vi "Trigger_CereStim_During_ PAL_Task.vi"() -> ()   [LabVIEW 2024]
uses:
  <vilib>/DAQmx/write.llb/DAQmx Write (Analog DBL 1Chan 1Samp).vi
  <vilib>/DAQmx/read.llb/DAQmx Read (Analog 1D Wfm NChan 1Samp).vi
  <vilib>/DAQmx/create/channels.llb/DAQmx Create Channel (AI-Voltage-Basic).vi
  <vilib>/DAQmx/create/channels.llb/DAQmx Create Channel (AO-Voltage-Basic).vi
  <vilib>/DAQmx/miscellaneous.llb/DAQmx Fill In Error Info.vi
  <vilib>/measure/mamon.llb/Trigger Detection for 1 Channel.vi
  <vilib>/measure/NI_MAPro.lvlib
panel:
  in  "Stimulation Offset\n(only for cond 10)":dbl=1.0
  out "Last STIMULATION ON Time":timestamp format="%<%.6X\n%x>T"
  in  "Acquisition Fs":i32=200
  in  "STIM 1 On 1 OFF":bool=TRUE
  out "Stimulation Pulse Counter":u64
  in  "Stimulation TTL Freq":dbl=50.0
  out "Reinforcement Threshold For Correct Incorrect":dbl
  in  "Reinforcement Signal Duration\nFor Incorrect":dbl=0.1
  in  "Reinforcement Signal Duration\nFor correct":dbl=0.07
  in  "Hysthersis":dbl=0.1
  in  "Event Detection Threshold (V)":dbl=3.0
  out "% NoSTIM Success":dbl format="%2_2g"
  out "#Success: NoSTIM":u32
  out "# Trials: NoSTIM":u32
  out "% STIM Success":dbl format="%2_2g"
  out "# Success: STIM":u32
  out "# Trials: STIM":u32
  out "% Success":dbl format="%2_2g"
  out "# Success":u32
  in  "Set StimulationManually, ALWAYS:":bool=TRUE
  in  "Manually Control Stimulation":bool=TRUE
  out "Trial Structure":string[](array[string])
  in  "Stimulation Probability":dbl=0.5 min=0.05 max=0.95 step=0.1
  out "Stimulation ON?":bool
  out "Time Elapsed since last event Offset":dbl
  out "Time Elapsed Since last trial":dbl
  out "Last STIMULUSINFO OFF":timestamp format="%<%.6X\n%x>T"
  out "Time Last Reinforcement":timestamp format="%<%.6X\n%x>T"
  out "Last Trial End":timestamp format="%<%.6X\n%x>T"
  out "Stimulation Trial":bool
  in  "Stimulation Onset time (Before each event )":dbl=2.0
  out "# Trials":u32
  out "Previous Trial: Correct/Incorrect":bool
  in  "STIMULATION CONDITION":u16(ring)=4 items=["--NONE SELECTED--", "1 Pre Sample Onset (STOPS AT STIMULUSINFO OFF)", "2 Pre Choice Onset (STOPS AT STIMULUSINFO OFF)", "3 Pre Sample And Choice Onset (STOPS AT STIMULUSINFO OFF)", "4 Pre 1st Sample till SamplePhase Offset ", "5 Pre 1st Choice till ChoicePhase Offset ", "6 During MemoryDelay  (NO STIMULATION ONSET TIME)", "7 During ITI (NO STIMULATION ONSET TIME)", "8 Entire Trial (Starts Pre 1st Sample ends at trial end)", "*9 Pre Sample Onset (STOPS AT STIMULUSINFO ON)", "10 PreStim(n-m seconds)"]
  out "ReinfoDur":dbl format="%_4g"
  out "TIME Reinforcement OFF":timestamp format="%<%.6X\n%x>T"
  out "TIME Reinforcement ON":timestamp format="%<%.6X\n%x>T"
  out "REINFORCEMENTINFO \nOFF Count":u32
  out "REINFORCEMENTINFO \nON Count":u32
  out "STIMULUSINFO \nOFF Count":u32
  out "STIMULUSINFO \nON Count":u32
  in  "stop":bool
  in  "Punishment Dur":dbl=7.0
  in  "Pump Dur":dbl=2.0
  in  "Memory Delay":dbl=7.0
  in  "Stimulation Fs":i32=1000
  in  "ITI":dbl=5.0
  in  "PAL TASK":u16=4
  in  "ICI":dbl=4.0
  in  "ISI":dbl=3.0
  # "PAL TASK"
  # "Tracking timings and events"
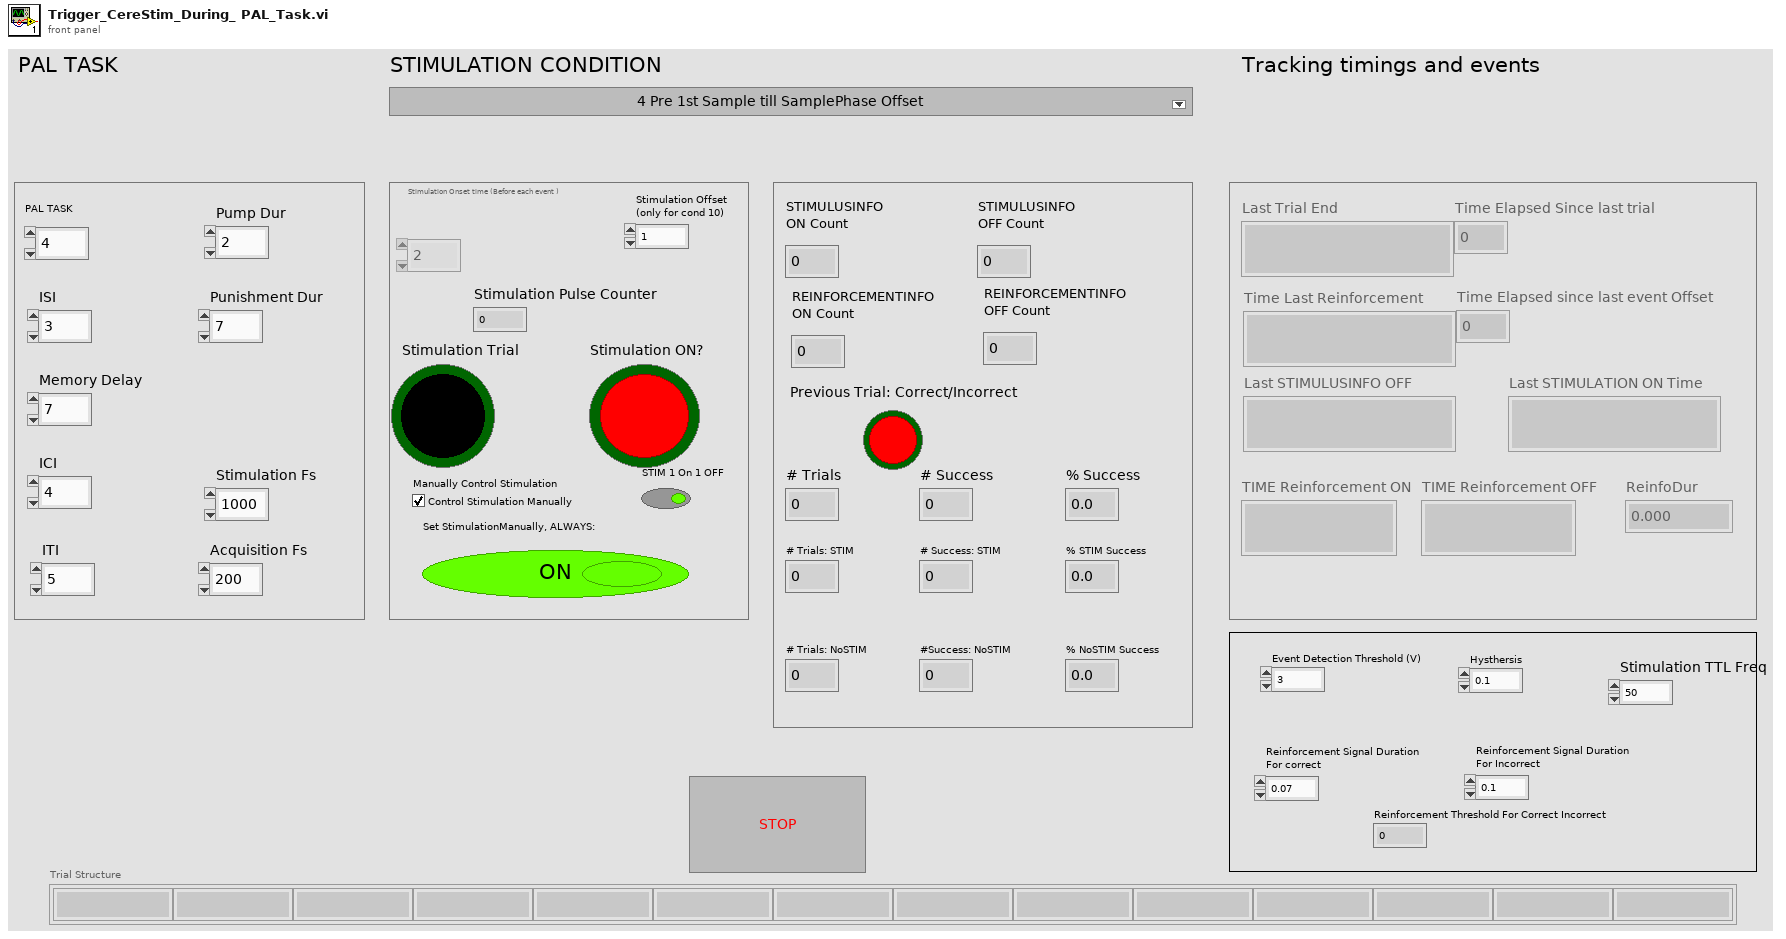
[diagram p1: front panel]
types:
  T1 = enum8{"Enabled", "Disabled", "Disabled and Grayed Out"}
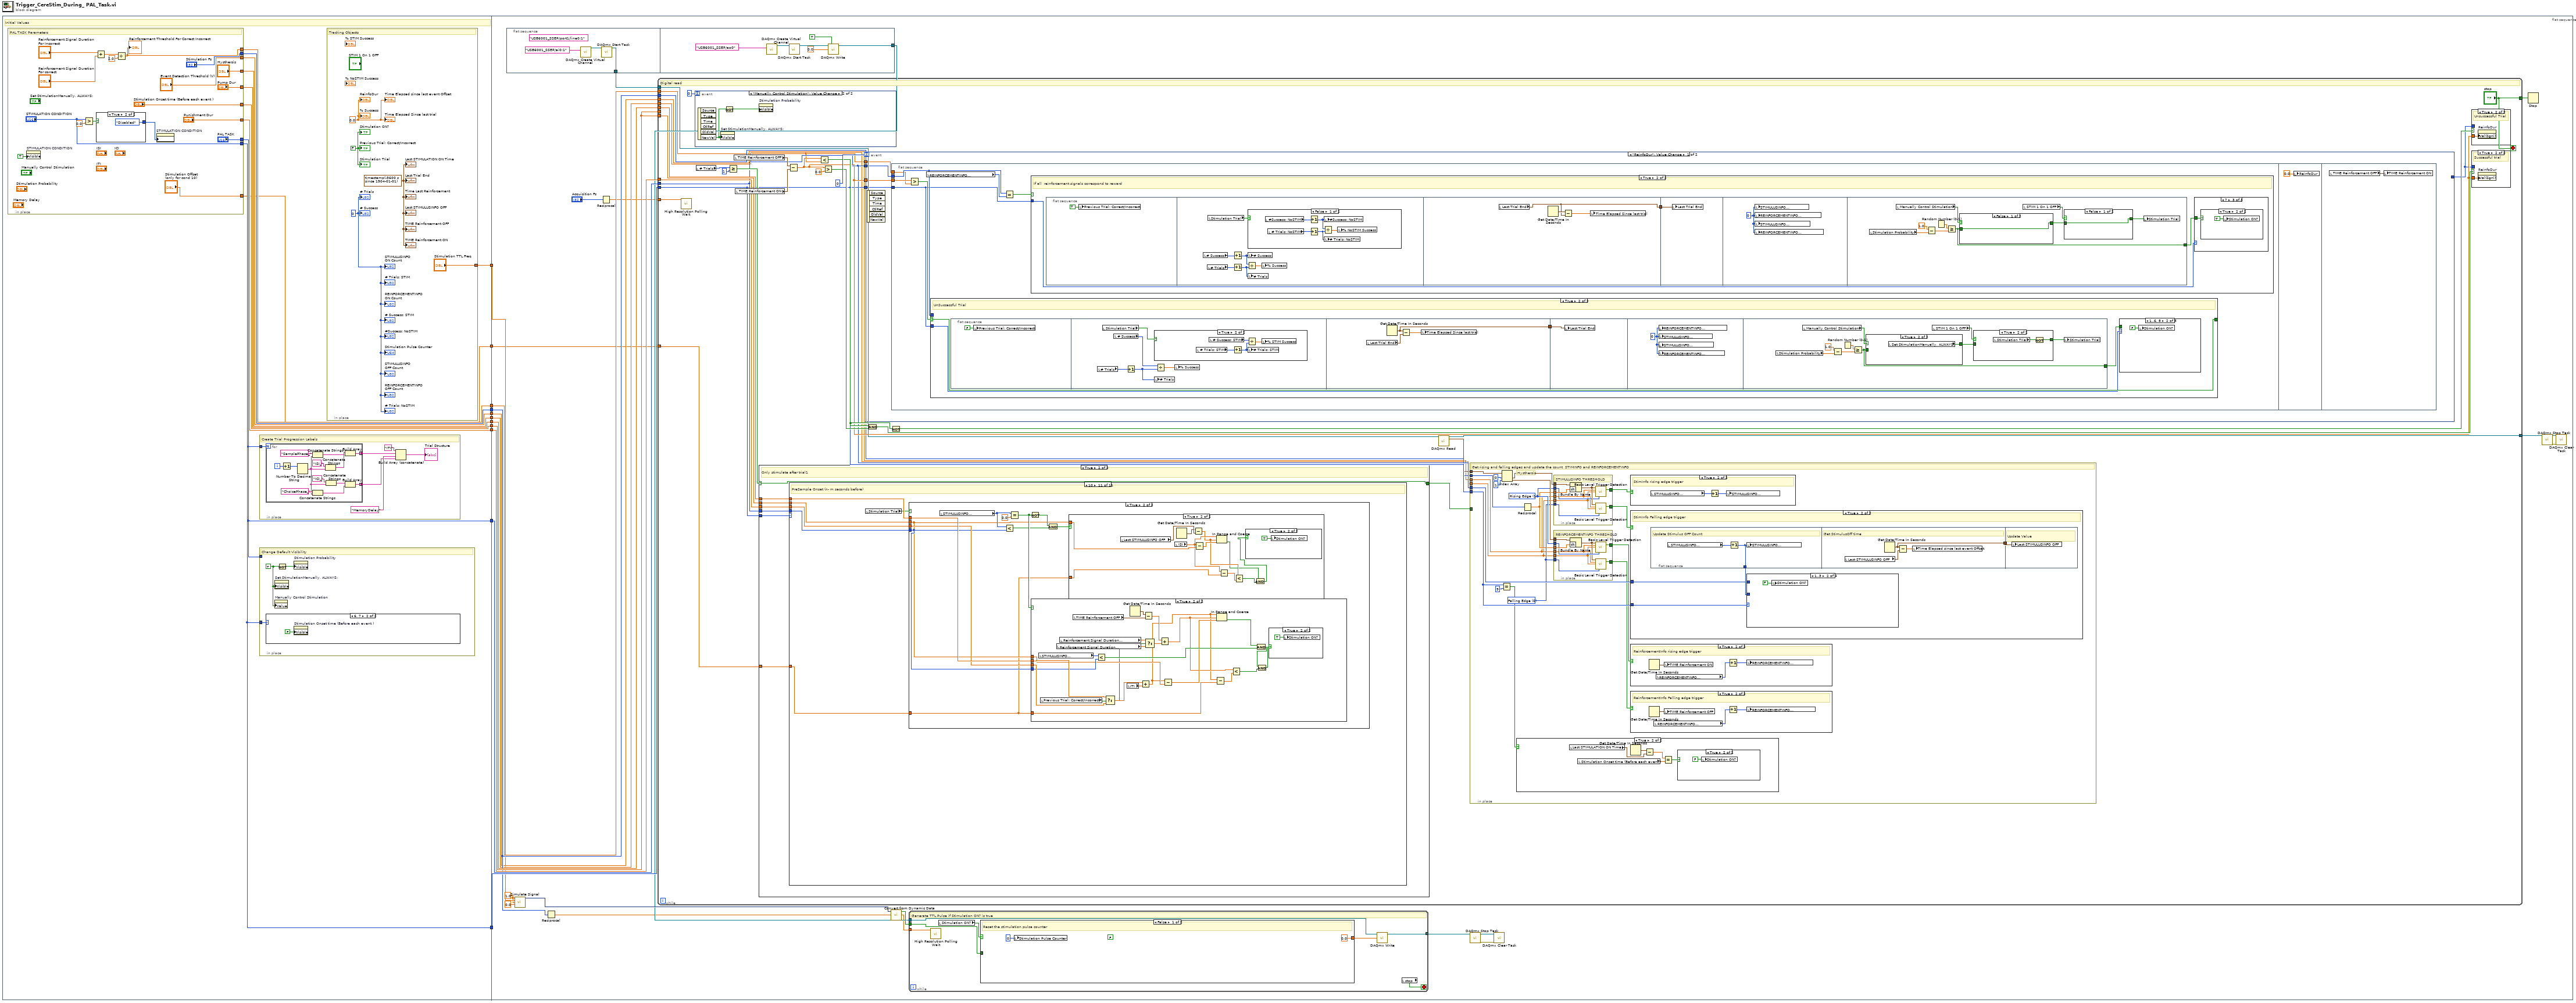
[diagram p0: block diagram]
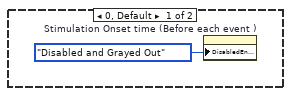
[diagram p2: hidden frame]
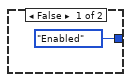
[diagram p3: hidden frame]
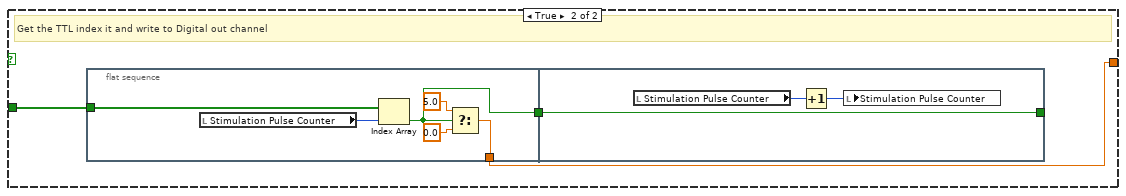
[diagram p4: hidden frame]
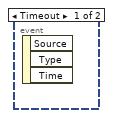
[diagram p5: hidden frame]
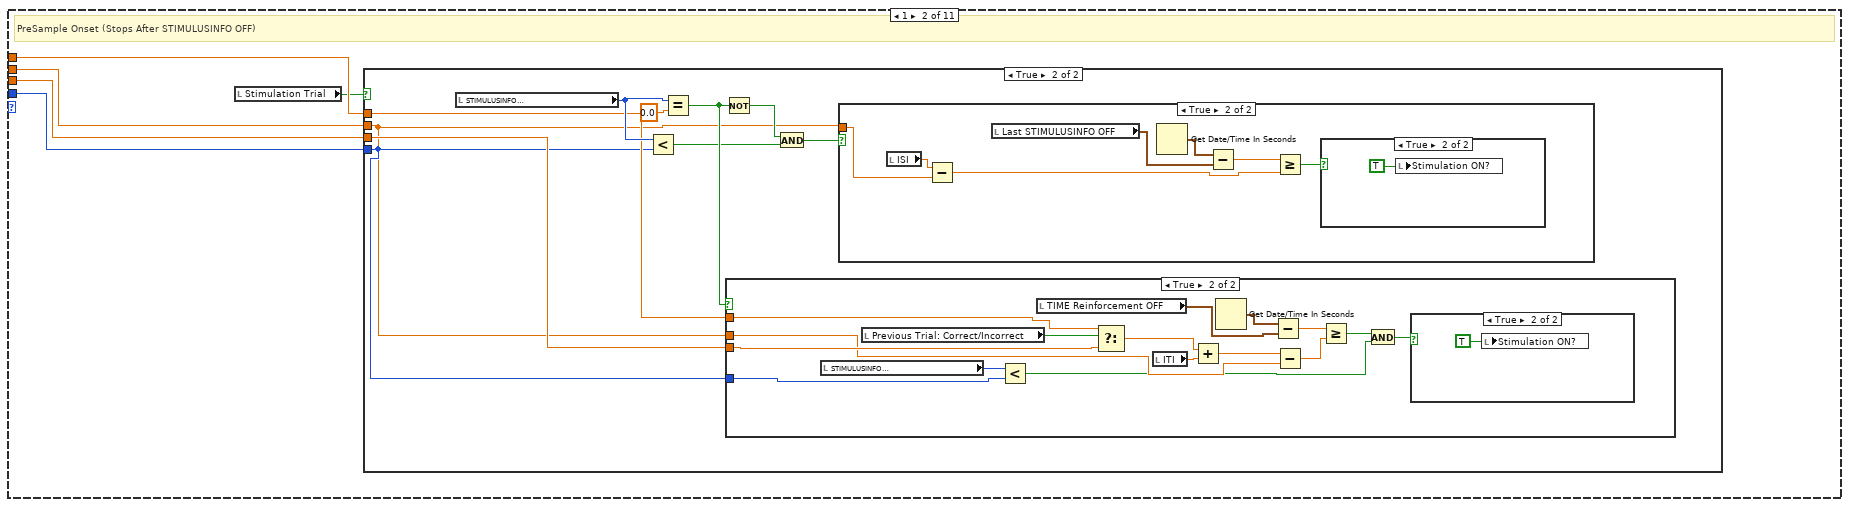
[diagram p8: hidden frame]
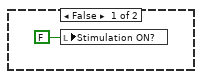
[diagram p13: hidden frame]
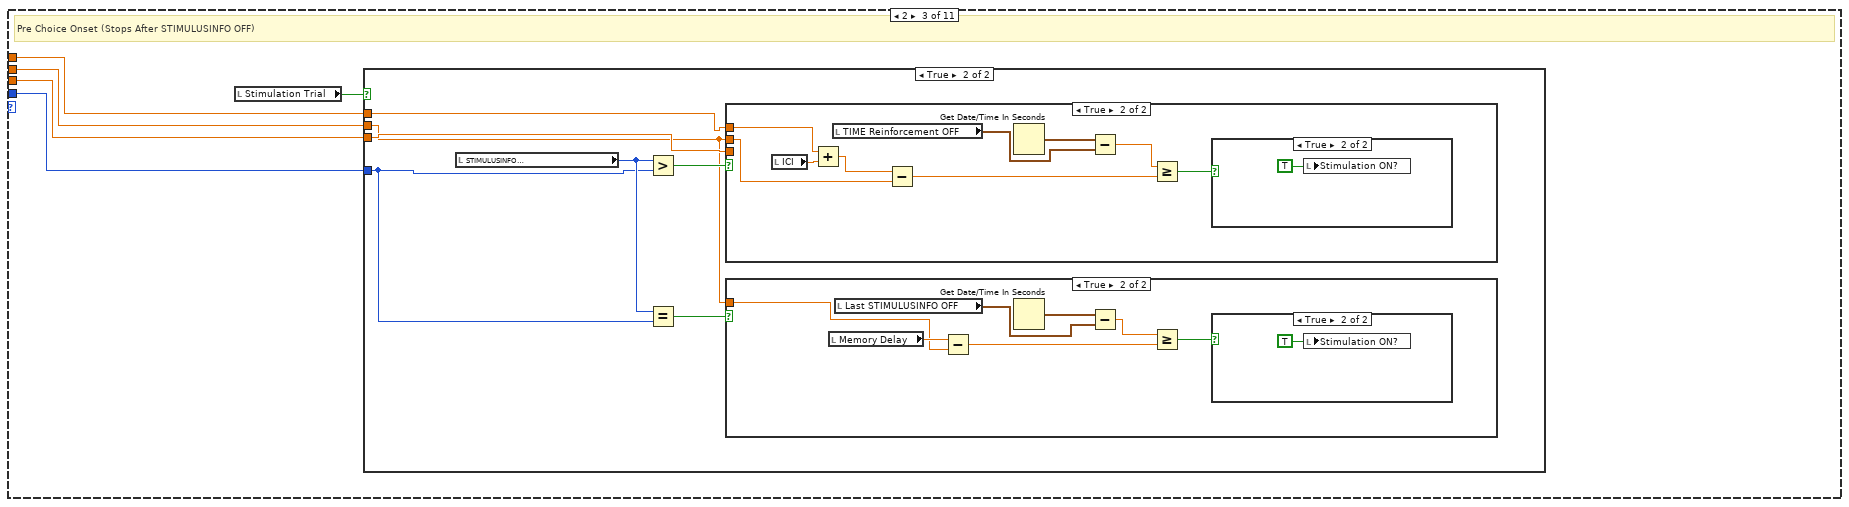
[diagram p14: hidden frame]
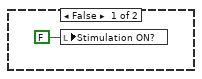
[diagram p19: hidden frame]
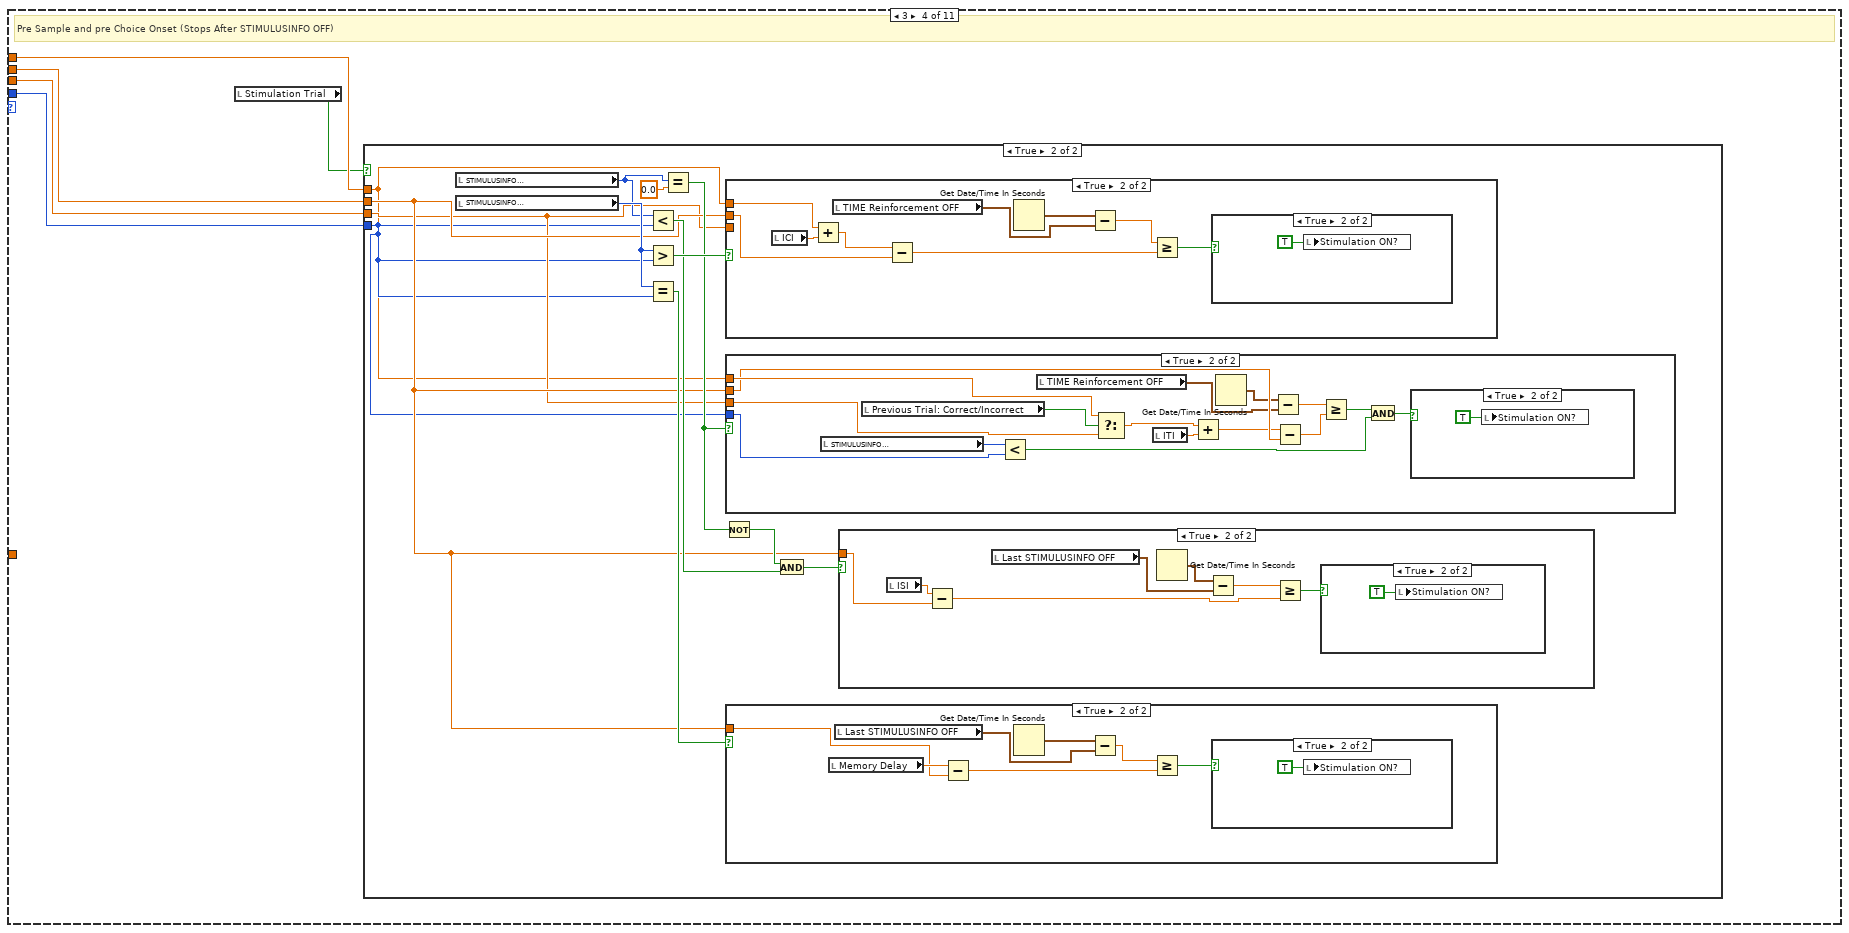
[diagram p20: hidden frame]
diagram:
  n1 = flat-sequence {
    tunnel: [w19] -> w11
    tunnel: [w20] -> w10
    tunnel: [w18] -> w9
    tunnel: [w22] -> w8
    tunnel: [w21] -> w7
    tunnel: [w17] -> w6
    tunnel: [w16] -> w5
    tunnel: [w15] -> w4
    tunnel: [w14] -> w3
    tunnel: [w13] -> w2
    tunnel: [w12] -> w1
    tunnel: w11 -> [w96]
    tunnel: w10 -> [w92]
    tunnel: w9 -> [w91]
    tunnel: w8 -> [w90]
    tunnel: w7 -> [w89]
    tunnel: w6 -> [w88]
    tunnel: w5 -> [w87]
    tunnel: w4 -> [w86]
    tunnel: w3 -> [w85]
    tunnel: w2 -> [w84]
    tunnel: w1 -> [w72]
    frame #0 {
      # "Initial Values"
      n2 = in-place {
        in-place-border: ["Stimulation Onset time (Before each event )"] -> w20
        in-place-border: ["PAL TASK"] -> w19
        in-place-border: ["Pump Dur"] -> w22
        in-place-border: ["Punishment Dur"] -> w21
        in-place-border: ["STIMULATION CONDITION"] -> w18
        in-place-border: ["Stimulation Fs"] -> w17
        in-place-border: ["Event Detection Threshold (V)"] -> w16
        in-place-border: ["Hysthersis"] -> w15
        in-place-border: [w58] -> w14
        in-place-border: ["Stimulation Offset\n(only for cond 10)"] -> w12
        # "PAL TASK Parameters"
        n3 = property on="STIMULATION CONDITION" class="Ring (strict)"("Visible"=TRUE) -> ()  [unwired: 2 in, 2 out]
        n4 = Greater?(x="STIMULATION CONDITION", y=0.0) -> (0:w57:bool)
        n5 = Add(x="Reinforcement Signal Duration\nFor Incorrect", y="Reinforcement Signal Duration\nFor correct") -> (x+y=w60:dbl)
        n6 = case shown="True" w57 {
          tunnel: [T1."Enabled" ("Disabled") T1."Disabled" ("Disabled")] -> w54
          frame False {
          }
          frame True {
          }
        }
        n7 = Divide(x=w60, y=2.0) -> (x/y=w58:dbl)
        "Reinforcement Threshold For Correct Incorrect" <- w58
        n8 = property on="STIMULATION CONDITION" class="Ring (strict)"("DisabledEnum"=w54) -> ()  [unwired: 2 in, 2 out]
      }
      n9 = in-place {
        in-place-border: w19 -> [w29]
        # "Create Trial Progression Labels"
        n10 = for {
          N: w29 -> [_]
          tunnel: [w39] -> w32 mode=concatenating
          tunnel: [w36] -> w30 mode=concatenating
          i -> [w34]
          n11 = Increment(x=w34) -> (x+1=w35:i32)
          n12 = Number To Decimal String(number=w35) -> (decimal integer string=w42:string)  [unwired: 1 in]
          n13 = Concatenate Strings("SamplePhase_", w42) -> (w40:string)
          n14 = Concatenate Strings("ChoicePhase_", w42) -> (w37:string)
          n15 = Concatenate Strings("ISI_", w42) -> (w41:string)
          n16 = Concatenate Strings("ICI_", w42) -> (w38:string)
          n17 = Build Array(w41, w40) -> (w39:string[])
          n18 = Build Array(w38, w37) -> (w36:string[])
        }
        n19 = Build Array (concatenate)("ITI", w32, "MemoryDelay", w30) -> (→"Trial Structure":string[])
      }
      n20 = in-place {
        in-place-border: w19 -> [_]
        in-place-border: w18 -> [w23]
        w25 = TRUE
        # "Change Default Visibility"
        n21 = case shown="6, 7" w23 {
          frame 0, Default {
            n22 = property on="Stimulation Onset time (Before each event )" class="DigNum (strict)"("DisabledEnum"=T1."Disabled and Grayed Out" ("Disabled")) -> ()  [unwired: 2 in, 2 out]
          }
          frame 6, 7 {
            n23 = property on="Stimulation Onset time (Before each event )" class="DigNum (strict)"("Visible"=FALSE) -> ()  [unwired: 2 in, 2 out]
          }
        }
        n24 = property on="Set StimulationManually, ALWAYS:" class="Bool (strict)"("Visible"=w25) -> ()  [unwired: 2 in, 2 out]
        n25 = property on="Manually Control Stimulation" class="Bool (strict)"("Value"=w25) -> ()  [unwired: 2 in, 2 out]
        n26 = Not(x=w25) -> (.not. x?=w24:bool)
        n27 = property on="Stimulation Probability" class="DigNum (strict)"("Visible"=w24) -> ()  [unwired: 2 in, 2 out]
      }
      n28 = in-place {
        in-place-border: ["Stimulation TTL Freq"] -> w13
        w50 = 0.0 ("ReinfoDur")
        w47 = timestamp(-3600 s since 1904-01-01) ("TIME Reinforcement ON")
        w51 = FALSE
        w48 = 0
        # "Tracking Objects"
        "STIMULUSINFO \nON Count" <- w48
        "REINFORCEMENTINFO \nON Count" <- w48
        "STIMULUSINFO \nOFF Count" <- w48
        "REINFORCEMENTINFO \nOFF Count" <- w48
        "# Trials" <- w48
        "Previous Trial: Correct/Incorrect" <- w51
        "Stimulation Trial" <- w51
        "Stimulation ON?" <- w51
        "TIME Reinforcement ON" <- w47
        "TIME Reinforcement OFF" <- w47
        "ReinfoDur" <- w50
        "Last Trial End" <- w47
        "Time Last Reinforcement" <- w47
        "Last STIMULUSINFO OFF" <- w47
        "Time Elapsed Since last trial" <- w50
        "Time Elapsed since last event Offset" <- w50
        "# Success" <- w48
        "% Success" <- w50
        "# Trials: STIM" <- w48
        "# Trials: NoSTIM" <- w48
        "# Success: STIM" <- w48
        "#Success: NoSTIM" <- w48
        "Stimulation Pulse Counter" <- w48
        "Last STIMULATION ON Time" <- w47
      }
    }
    frame #1 {
      w83 = 1.0 ("Amplitude")
      n29 = flat-sequence {
        tunnel: [w121] -> w93
        tunnel: [w125] -> w79
        frame #0 {
          (unwired) tag "USB6001_SSEP/port1/line0:1" ("lines")
          n30 = call-poly <vilib>:"DAQmx Create Virtual Channel.vi"("physical channels"=tag "USB6001_SSEP/ai0:1") -> ("task out"=w122:refnum<k21>)  [unwired: 13 in, 1 out]
          n31 = call <vilib>:"DAQmx Start Task.vi"("task/channels in"=w122) -> ("task out"=w121:refnum<k21>)  [unwired: 13 in, 1 out]
        }
        frame #1 {
          n32 = call-poly <vilib>:"DAQmx Create Virtual Channel.vi"("physical channels"=tag "USB6001_SSEP/ao0") -> ("task out"=w127:refnum<k21>)  [unwired: 13 in, 1 out]
          n33 = call <vilib>:"DAQmx Start Task.vi"("task/channels in"=w127) -> ("task out"=w128:refnum<k21>)  [unwired: 13 in, 1 out]
          n34 = call-poly <vilib>:"DAQmx Write.vi"("task/channels in"=w128, "auto start"=TRUE, "data"=0.0) -> ("task out"=w125:refnum<k21>)  [unwired: 10 in, 2 out]
        }
      }
      n35 = call "Simulate Signal"("Offset"=w83, "Frequency"=w84, "Amplitude"=w83, "Phase"=0.0) -> ("TTL STIMULATION SIG"=w81:dynamicdata)  [unwired: 10 in, 1 out]
      n36 = Reciprocal(x=w88) -> (1/x=w73:dbl)
      n37 = Reciprocal(x="Acquisition Fs") -> (1/x=w74:dbl)
      n38 = while {
        tunnel: w93 -> [w158]
        tunnel: [w157] -> w97
        tunnel: w96 -> [w139]
        tunnel: ["stop"] -> w94
        tunnel: w91 -> [w137]
        tunnel: w92 -> [w142]
        tunnel: w92 -> [_]
        tunnel: w90 -> [w141]
        tunnel: w89 -> [w140]
        tunnel: w88 -> [w134]
        tunnel: w87 -> [w133]
        tunnel: w86 -> [w132]
        tunnel: w85 -> [w131]
        tunnel: w74 -> [w130]
        tunnel: w72 -> [w129]
        stop <- "stop" stop-if-true
        # "Digital read"
        n39 = call <vilib>:"High Resolution Polling Wait.vi"("seconds to wait"=w130) -> ()  [unwired: 10 in, 1 out]
        n40 = event shown="[1] \"Manually Control Stimulation\": Value Change" {
          selector: _ -> [_ _]
          dyn-events: _ -> [_ _]
          timeout: 0 -> [_ _]
          event Timeout {
            n41 = event-data() -> ()  [unwired: 1 in, 3 out]
          }
          event "Manually Control Stimulation": Value Change {
            n42 = event-data() -> ("NewVal"=w159:bool)  [unwired: 1 in, 5 out]
            n43 = property on="Set StimulationManually, ALWAYS:" class="Bool (strict)"("Visible"=w159) -> ()  [unwired: 2 in, 2 out]
            n44 = Not(x=w159) -> (.not. x?=w160:bool)
            n45 = property on="Stimulation Probability" class="DigNum (strict)"("Visible"=w160) -> ()  [unwired: 2 in, 2 out]
          }
        }
        n46 = local read "# Trials"() -> (w145:u32)
        n47 = Greater Or Equal?(x=w145, y=u32 1) -> (x >= y?=w143:bool)
        n48 = local read "TIME Reinforcement OFF"() -> (w155:timestamp)
        n49 = local read "TIME Reinforcement ON"() -> (w156:timestamp)
        n50 = case shown="True" w143 {
          selector: w143 -> [w161 w163]
          tunnel: w137 -> [_ w168]
          tunnel: w142 -> [_ w167]
          tunnel: w139 -> [_ w166]
          tunnel: w141 -> [_ w165]
          tunnel: w140 -> [_ w164]
          tunnel: [w161 w163] -> w138
          tunnel: w129 -> [_ w162]
          frame False {
          }
          frame True {
            # "Only stimulate after trial1"
            n51 = case shown="10" w168 {
              tunnel: w167 -> [_ w170 w211 w245 w308 w335 _ _ w367 w387 w434]
              tunnel: w166 -> [_ w171 w214 w243 w306 w334 w354 _ w368 w388 w435]
              tunnel: w165 -> [_ w173 w213 w242 w305 _ _ _ w365 w390 w437]
              tunnel: w164 -> [_ w172 w212 w244 w307 _ _ _ w366 w389 w436]
              tunnel: w162 -> [_ _ _ _ _ _ _ _ _ _ w432]
              frame 0, Default {
              }
              frame 1 {
                # "PreSample Onset (Stops After STIMULUSINFO OFF)"
                n52 = local read "Stimulation Trial"() -> (w169:bool)
                n53 = case shown="True" w169 {
                  tunnel: w173 -> [_ w178]
                  tunnel: w172 -> [_ w177]
                  tunnel: w171 -> [_ w175]
                  tunnel: w170 -> [_ w174]
                  frame False {
                  }
                  frame True {
                    n54 = local read "STIMULUSINFO \nOFF Count"() -> (w181:u32)
                    n55 = Less?(x=w181, y=w175) -> (x < y?=w179:bool)
                    n56 = Equal?(x=w181, y=0.0) -> (x = y?=w182:bool)
                    n57 = Not(x=w182) -> (.not. x?=w183:bool)
                    n58 = case shown="True" w182 {
                      tunnel: w178 -> [_ w199]
                      tunnel: w177 -> [_ w198]
                      tunnel: w175 -> [_ w197]
                      tunnel: w174 -> [_ w196]
                      frame False {
                      }
                      frame True {
                        n59 = local read "STIMULUSINFO \nOFF Count"() -> (w188:u32)
                        n60 = local read "Previous Trial: Correct/Incorrect"() -> (w187:bool)
                        n61 = Less?(x=w188, y=w197) -> (x < y?=w190:bool)
                        n62 = local read "TIME Reinforcement OFF"() -> (w194:timestamp)
                        n63 = Select(t=w199, s=w187, f=w198) -> (s? t:f=w186:dbl)
                        n64 = local read "ITI"() -> (w185:dbl)
                        n65 = Add(x=w186, y=w185) -> (x+y=w184:dbl)
                        n66 = Get Date/Time In Seconds() -> (seconds since 1Jan1904=w195:timestamp)
                        n67 = Subtract(x=w195, y=w194) -> (x-y=w193:dbl)
                        n68 = Subtract(x=w184, y=w196) -> (x-y=w192:dbl)
                        n69 = Greater Or Equal?(x=w193, y=w192) -> (x >= y?=w191:bool)
                        n70 = And(x=w191, y=w190) -> (x .and. y?=w189:bool)
                        n71 = case shown="True" w189 {
                          frame False {
                          }
                          frame True {
                            n72 = local write "Stimulation ON?"(TRUE ("Stimulation ON?")) -> ()
                          }
                        }
                      }
                    }
                    n73 = And(x=w183, y=w179) -> (x .and. y?=w180:bool)
                    n74 = case shown="True" w180 {
                      tunnel: w174 -> [_ w201]
                      frame False {
                      }
                      frame True {
                        n75 = local read "ISI"() -> (w204:dbl)
                        n76 = Subtract(x=w204, y=w201) -> (x-y=w206:dbl)
                        n77 = local read "Last STIMULUSINFO OFF"() -> (w203:timestamp)
                        n78 = Get Date/Time In Seconds() -> (seconds since 1Jan1904=w202:timestamp)
                        n79 = Subtract(x=w202, y=w203) -> (x-y=w205:dbl)
                        n80 = Greater Or Equal?(x=w205, y=w206) -> (x >= y?=w207:bool)
                        n81 = case shown="True" w207 {
                          frame False {
                            n82 = local write "Stimulation ON?"(FALSE ("Stimulation ON?")) -> ()
                          }
                          frame True {
                            n83 = local write "Stimulation ON?"(TRUE ("Stimulation ON?")) -> ()
                          }
                        }
                      }
                    }
                  }
                }
              }
              frame 2 {
                # "Pre Choice Onset (Stops After STIMULUSINFO OFF)"
                n84 = local read "Stimulation Trial"() -> (w210:bool)
                n85 = case shown="True" w210 {
                  tunnel: w214 -> [_ w216]
                  tunnel: w213 -> [_ w218]
                  tunnel: w212 -> [_ w217]
                  tunnel: w211 -> [_ w215]
                  frame False {
                  }
                  frame True {
                    n86 = local read "STIMULUSINFO \nOFF Count"() -> (w219:u32)
                    n87 = Greater?(x=w219, y=w216) -> (0:w220:bool)
                    n88 = Equal?(x=w219, y=w216) -> (x = y?=w221:bool)
                    n89 = case shown="True" w220 {
                      tunnel: w218 -> [_ w222]
                      tunnel: w217 -> [_ _]
                      tunnel: w215 -> [_ w230]
                      frame False {
                      }
                      frame True {
                        n90 = local read "ICI"() -> (w224:dbl)
                        n91 = Add(x=w222, y=w224) -> (x+y=w223:dbl)
                        n92 = local read "TIME Reinforcement OFF"() -> (w228:timestamp)
                        n93 = Subtract(x=w223, y=w230) -> (x-y=w226:dbl)
                        n94 = Get Date/Time In Seconds() -> (seconds since 1Jan1904=w229:timestamp)
                        n95 = Subtract(x=w229, y=w228) -> (x-y=w227:dbl)
                        n96 = Greater Or Equal?(x=w227, y=w226) -> (x >= y?=w225:bool)
                        n97 = case shown="True" w225 {
                          frame False {
                          }
                          frame True {
                            n98 = local write "Stimulation ON?"(TRUE ("Stimulation ON?")) -> ()
                          }
                        }
                      }
                    }
                    n99 = case shown="True" w221 {
                      tunnel: w215 -> [_ w232]
                      frame False {
                      }
                      frame True {
                        n100 = local read "Memory Delay"() -> (w235:dbl)
                        n101 = local read "Last STIMULUSINFO OFF"() -> (w234:timestamp)
                        n102 = Subtract(x=w235, y=w232) -> (x-y=w237:dbl)
                        n103 = Get Date/Time In Seconds() -> (seconds since 1Jan1904=w233:timestamp)
                        n104 = Subtract(x=w233, y=w234) -> (x-y=w236:dbl)
                        n105 = Greater Or Equal?(x=w236, y=w237) -> (x >= y?=w238:bool)
                        n106 = case shown="True" w238 {
                          frame False {
                            n107 = local write "Stimulation ON?"(FALSE ("Stimulation ON?")) -> ()
                          }
                          frame True {
                            n108 = local write "Stimulation ON?"(TRUE ("Stimulation ON?")) -> ()
                          }
                        }
                      }
                    }
                  }
                }
              }
              frame 3 {
                # "Pre Sample and pre Choice Onset (Stops After STIMULUSINFO OFF)"
                n109 = local read "Stimulation Trial"() -> (w241:bool)
                n110 = case shown="True" w241 {
                  tunnel: w245 -> [_ w249]
                  tunnel: w244 -> [_ w248]
                  tunnel: w243 -> [_ w247]
                  tunnel: w242 -> [_ w246]
                  frame False {
                  }
                  frame True {
                    n111 = local read "STIMULUSINFO \nOFF Count"() -> (w253:u32)
                    n112 = local read "STIMULUSINFO \nOFF Count"() -> (w258:u32)
                    n113 = Less?(x=w253, y=w247) -> (x < y?=w255:bool)
                    n114 = Greater?(x=w258, y=w247) -> (0:w257:bool)
                    n115 = Equal?(x=w258, y=w247) -> (x = y?=w256:bool)
                    n116 = Equal?(x=w253, y=0.0) -> (x = y?=w251:bool)
                    n117 = Not(x=w251) -> (.not. x?=w250:bool)
                    n118 = case shown="True" w257 {
                      tunnel: w246 -> [_ w285]
                      tunnel: w248 -> [_ _]
                      tunnel: w249 -> [_ w293]
                      frame False {
                      }
                      frame True {
                        n119 = local read "ICI"() -> (w287:dbl)
                        n120 = Add(x=w285, y=w287) -> (x+y=w286:dbl)
                        n121 = local read "TIME Reinforcement OFF"() -> (w291:timestamp)
                        n122 = Subtract(x=w286, y=w293) -> (x-y=w289:dbl)
                        n123 = Get Date/Time In Seconds() -> (seconds since 1Jan1904=w292:timestamp)
                        n124 = Subtract(x=w292, y=w291) -> (x-y=w290:dbl)
                        n125 = Greater Or Equal?(x=w290, y=w289) -> (x >= y?=w288:bool)
                        n126 = case shown="True" w288 {
                          frame False {
                          }
                          frame True {
                            n127 = local write "Stimulation ON?"(TRUE ("Stimulation ON?")) -> ()
                          }
                        }
                      }
                    }
                    n128 = case shown="True" w251 {
                      tunnel: w246 -> [_ w274]
                      tunnel: w248 -> [_ w273]
                      tunnel: w247 -> [_ w272]
                      tunnel: w249 -> [_ w271]
                      frame False {
                      }
                      frame True {
                        n129 = local read "STIMULUSINFO \nOFF Count"() -> (w263:u32)
                        n130 = local read "Previous Trial: Correct/Incorrect"() -> (w262:bool)
                        n131 = Less?(x=w263, y=w272) -> (x < y?=w265:bool)
                        n132 = local read "TIME Reinforcement OFF"() -> (w269:timestamp)
                        n133 = Select(t=w274, s=w262, f=w273) -> (s? t:f=w261:dbl)
                        n134 = local read "ITI"() -> (w260:dbl)
                        n135 = Add(x=w261, y=w260) -> (x+y=w259:dbl)
                        n136 = Get Date/Time In Seconds() -> (seconds since 1Jan1904=w270:timestamp)
                        n137 = Subtract(x=w270, y=w269) -> (x-y=w268:dbl)
                        n138 = Subtract(x=w259, y=w271) -> (x-y=w267:dbl)
                        n139 = Greater Or Equal?(x=w268, y=w267) -> (x >= y?=w266:bool)
                        n140 = And(x=w266, y=w265) -> (x .and. y?=w264:bool)
                        n141 = case shown="True" w264 {
                          frame False {
                          }
                          frame True {
                            n142 = local write "Stimulation ON?"(TRUE ("Stimulation ON?")) -> ()
                          }
                        }
                      }
                    }
                    n143 = case shown="True" w256 {
                      tunnel: w249 -> [_ w295]
                      frame False {
                      }
                      frame True {
                        n144 = local read "Memory Delay"() -> (w298:dbl)
                        n145 = local read "Last STIMULUSINFO OFF"() -> (w297:timestamp)
                        n146 = Subtract(x=w298, y=w295) -> (x-y=w300:dbl)
                        n147 = Get Date/Time In Seconds() -> (seconds since 1Jan1904=w296:timestamp)
                        n148 = Subtract(x=w296, y=w297) -> (x-y=w299:dbl)
                        n149 = Greater Or Equal?(x=w299, y=w300) -> (x >= y?=w301:bool)
                        n150 = case shown="True" w301 {
                          frame False {
                            n151 = local write "Stimulation ON?"(FALSE ("Stimulation ON?")) -> ()
                          }
                          frame True {
                            n152 = local write "Stimulation ON?"(TRUE ("Stimulation ON?")) -> ()
                          }
                        }
                      }
                    }
                    n153 = And(x=w250, y=w255) -> (x .and. y?=w254:bool)
                    n154 = case shown="True" w254 {
                      tunnel: w249 -> [_ w276]
                      frame False {
                      }
                      frame True {
                        n155 = local read "ISI"() -> (w279:dbl)
                        n156 = Subtract(x=w279, y=w276) -> (x-y=w281:dbl)
                        n157 = local read "Last STIMULUSINFO OFF"() -> (w278:timestamp)
                        n158 = Get Date/Time In Seconds() -> (seconds since 1Jan1904=w277:timestamp)
                        n159 = Subtract(x=w277, y=w278) -> (x-y=w280:dbl)
                        n160 = Greater Or Equal?(x=w280, y=w281) -> (x >= y?=w282:bool)
                        n161 = case shown="True" w282 {
                          frame False {
                            n162 = local write "Stimulation ON?"(FALSE ("Stimulation ON?")) -> ()
                          }
                          frame True {
                            n163 = local write "Stimulation ON?"(TRUE ("Stimulation ON?")) -> ()
                          }
                        }
                      }
                    }
                  }
                }
              }
              frame 4 {
                # "Pre Sample till SamplePhase is over"
                n164 = local read "Stimulation Trial"() -> (w304:bool)
                n165 = case shown="True" w304 {
                  tunnel: w308 -> [_ w312]
                  tunnel: w307 -> [_ w311]
                  tunnel: w306 -> [_ w310]
                  tunnel: w305 -> [_ w309]
                  frame False {
                  }
                  frame True {
                    n166 = local read "STIMULUSINFO \nOFF Count"() -> (w315:u32)
                    n167 = Equal?(x=w315, y=0.0) -> (x = y?=w313:bool)
                    n168 = case shown="True" w313 {
                      tunnel: w309 -> [_ w331]
                      tunnel: w311 -> [_ w330]
                      tunnel: w310 -> [_ w329]
                      tunnel: w312 -> [_ w328]
                      frame False {
                      }
                      frame True {
                        n169 = local read "STIMULUSINFO \nOFF Count"() -> (w320:u32)
                        n170 = local read "Previous Trial: Correct/Incorrect"() -> (w319:bool)
                        n171 = Less?(x=w320, y=w329) -> (x < y?=w322:bool)
                        n172 = local read "TIME Reinforcement OFF"() -> (w326:timestamp)
                        n173 = Select(t=w331, s=w319, f=w330) -> (s? t:f=w318:dbl)
                        n174 = local read "ITI"() -> (w317:dbl)
                        n175 = Add(x=w318, y=w317) -> (x+y=w316:dbl)
                        n176 = Get Date/Time In Seconds() -> (seconds since 1Jan1904=w327:timestamp)
                        n177 = Subtract(x=w327, y=w326) -> (x-y=w325:dbl)
                        n178 = Subtract(x=w316, y=w328) -> (x-y=w324:dbl)
                        n179 = Greater Or Equal?(x=w325, y=w324) -> (x >= y?=w323:bool)
                        n180 = And(x=w323, y=w322) -> (x .and. y?=w321:bool)
                        n181 = case shown="True" w321 {
                          frame False {
                          }
                          frame True {
                            n182 = local write "Stimulation ON?"(TRUE ("Stimulation ON?")) -> ()
                          }
                        }
                      }
                    }
                  }
                }
              }
              frame 5 {
                # "Pre ChoicePhase till ChoicePhase is over"
                n183 = local read "Stimulation Trial"() -> (w333:bool)
                n184 = case shown="True" w333 {
                  tunnel: w335 -> [_ w337]
                  tunnel: w334 -> [_ w336]
                  frame False {
                  }
                  frame True {
                    n185 = local read "STIMULUSINFO \nOFF Count"() -> (w339:u32)
                    n186 = Equal?(x=w339, y=w336) -> (x = y?=w338:bool)
                    n187 = case shown="True" w338 {
                      tunnel: w337 -> [_ w340]
                      frame False {
                      }
                      frame True {
                        n188 = local read "Memory Delay"() -> (w343:dbl)
                        n189 = local read "Last STIMULUSINFO OFF"() -> (w342:timestamp)
                        n190 = Subtract(x=w343, y=w340) -> (x-y=w345:dbl)
                        n191 = Get Date/Time In Seconds() -> (seconds since 1Jan1904=w341:timestamp)
                        n192 = Subtract(x=w341, y=w342) -> (x-y=w344:dbl)
                        n193 = Greater Or Equal?(x=w344, y=w345) -> (x >= y?=w346:bool)
                        n194 = case shown="True" w346 {
                          frame False {
                            n195 = local write "Stimulation ON?"(FALSE ("Stimulation ON?")) -> ()
                          }
                          frame True {
                            n196 = local write "Stimulation ON?"(TRUE ("Stimulation ON?")) -> ()
                          }
                        }
                      }
                    }
                  }
                }
              }
              frame 6 {
                # "During MemoryDelay (NO StimulationOnset time)"
                n197 = local read "STIMULUSINFO \nOFF Count"() -> (w353:u32)
                n198 = local read "Stimulation Trial"() -> (w349:bool)
                n199 = local read "STIMULUSINFO \nON Count"() -> (w352:u32)
                n200 = case shown="True" w349 {
                  tunnel: w354 -> [_ w357]
                  tunnel: w353 -> [_ w355]
                  frame False {
                  }
                  frame True {
                    n201 = Equal?(x=w357, y=w355) -> (x = y?=w356:bool)
                    n202 = case shown="True" w356 {
                      frame False {
                      }
                      frame True {
                        n203 = local write "Stimulation ON?"(TRUE ("Stimulation ON?")) -> ()
                      }
                    }
                  }
                }
                n204 = Increment(x=w353) -> (x+1=w351:u32)
                n205 = Equal?(x=w351, y=w352) -> (x = y?=w350:bool)
                n206 = case shown="True" w350 {
                  frame False {
                  }
                  frame True {
                    n207 = local write "Stimulation ON?"(FALSE ("Stimulation ON?")) -> ()
                  }
                }
              }
              frame 7 {
                # "During ITI"
                n208 = local read "STIMULUSINFO \nON Count"() -> (w362:u32)
                n209 = Equal?(x=w362, y=u32 1) -> (x = y?=w360:bool)
                n210 = case shown="True" w360 {
                  frame False {
                  }
                  frame True {
                    n211 = local write "Stimulation ON?"(FALSE ("Stimulation ON?")) -> ()
                  }
                }
              }
              frame 8 {
                n212 = local read "Stimulation Trial"() -> (w364:bool)
                n213 = case shown="True" w364 {
                  tunnel: w368 -> [_ w372]
                  tunnel: w367 -> [_ w371]
                  tunnel: w366 -> [_ w370]
                  tunnel: w365 -> [_ w369]
                  frame False {
                  }
                  frame True {
                    n214 = local read "STIMULUSINFO \nOFF Count"() -> (w378:u32)
                    n215 = local read "Previous Trial: Correct/Incorrect"() -> (w377:bool)
                    n216 = Less?(x=w378, y=w372) -> (x < y?=w380:bool)
                    n217 = local read "TIME Reinforcement OFF"() -> (w373:timestamp)
                    n218 = Select(t=w369, s=w377, f=w370) -> (s? t:f=w376:dbl)
                    n219 = local read "ITI"() -> (w375:dbl)
                    n220 = Add(x=w376, y=w375) -> (x+y=w374:dbl)
                    n221 = Get Date/Time In Seconds() -> (seconds since 1Jan1904=w384:timestamp)
                    n222 = Subtract(x=w384, y=w373) -> (x-y=w383:dbl)
                    n223 = Subtract(x=w374, y=w371) -> (x-y=w382:dbl)
                    n224 = Greater Or Equal?(x=w383, y=w382) -> (x >= y?=w381:bool)
                    n225 = And(x=w381, y=w380) -> (x .and. y?=w379:bool)
                    n226 = case shown="True" w379 {
                      frame False {
                      }
                      frame True {
                        n227 = local write "Stimulation ON?"(TRUE ("Stimulation ON?")) -> ()
                      }
                    }
                  }
                }
              }
              frame 9 {
                # "PreSample Onset (Stops After STIMULUSINFO ON)"
                n228 = local read "Stimulation Trial"() -> (w386:bool)
                n229 = case shown="True" w386 {
                  tunnel: w390 -> [_ w395]
                  tunnel: w389 -> [_ w394]
                  tunnel: w388 -> [_ w392]
                  tunnel: w387 -> [_ w391]
                  frame False {
                  }
                  frame True {
                    n230 = local read "STIMULUSINFO \nOFF Count"() -> (w398:u32)
                    n231 = Less?(x=w398, y=w392) -> (x < y?=w396:bool)
                    n232 = Equal?(x=w398, y=0.0) -> (x = y?=w399:bool)
                    n233 = Not(x=w399) -> (.not. x?=w400:bool)
                    n234 = case shown="True" w399 {
                      tunnel: w395 -> [_ w420]
                      tunnel: w394 -> [_ w419]
                      tunnel: w392 -> [_ w418]
                      tunnel: w391 -> [_ w417]
                      frame False {
                      }
                      frame True {
                        n235 = local read "STIMULUSINFO \nOFF Count"() -> (w414:u32)
                        n236 = local read "Previous Trial: Correct/Incorrect"() -> (w406:bool)
                        n237 = local read "Reinforcement Signal Duration\nFor Incorrect"() -> (w405:dbl)
                        n238 = local read "Reinforcement Signal Duration\nFor correct"() -> (w404:dbl)
                        n239 = local read "TIME Reinforcement OFF"() -> (w416:timestamp)
                        n240 = Less?(x=w414, y=w418) -> (x < y?=w415:bool)
                        n241 = Select(t=w420, s=w406, f=w419) -> (s? t:f=w413:dbl)
                        n242 = local read "ITI"() -> (w412:dbl)
                        n243 = Get Date/Time In Seconds() -> (seconds since 1Jan1904=w411:timestamp)
                        n244 = Add(x=w413, y=w412) -> (x+y=w409:dbl)
                        n245 = Subtract(x=w411, y=w416) -> (x-y=w403:dbl)
                        n246 = Select(t=w404, s=w406, f=w405) -> (s? t:f=w401:dbl)
                        n247 = Subtract(x=w409, y=w417) -> (x-y=w408:dbl)
                        n248 = Add(x=w403, y=w401) -> (x+y=w402:dbl)
                        n249 = In Range and Coerce(upper limit=w409, x=w402, lower limit=w408) -> (In Range?=w407:bool)  [unwired: 1 out]
                        n250 = And(x=w407, y=w415) -> (x .and. y?=w410:bool)
                        n251 = case shown="True" w410 {
                          frame False {
                            n252 = local write "Stimulation ON?"(FALSE ("Stimulation ON?")) -> ()
                          }
                          frame True {
                            n253 = local write "Stimulation ON?"(TRUE ("Stimulation ON?")) -> ()
                          }
                        }
                      }
                    }
                    n254 = And(x=w400, y=w396) -> (x .and. y?=w397:bool)
                    n255 = case shown="True" w397 {
                      tunnel: w391 -> [_ w427]
                      frame False {
                      }
                      frame True {
                        n256 = local read "Last STIMULUSINFO OFF"() -> (w429:timestamp)
                        n257 = local read "ISI"() -> (w425:dbl)
                        n258 = Get Date/Time In Seconds() -> (seconds since 1Jan1904=w428:timestamp)
                        n259 = Subtract(x=w428, y=w429) -> (x-y=w426:dbl)
                        n260 = Subtract(x=w425, y=w427) -> (x-y=w424:dbl)
                        n261 = In Range and Coerce(upper limit=w425, x=w426, lower limit=w424) -> (In Range?=w423:bool)  [unwired: 1 out]
                        n262 = case shown="True" w423 {
                          frame False {
                            n263 = local write "Stimulation ON?"(FALSE ("Stimulation ON?")) -> ()
                          }
                          frame True {
                            n264 = local write "Stimulation ON?"(TRUE ("Stimulation ON?")) -> ()
                          }
                        }
                      }
                    }
                  }
                }
              }
              frame 10 {
                # "PreSample Onset (n- m seconds before)"
                n265 = local read "Stimulation Trial"() -> (w433:bool)
                n266 = case shown="True" w433 {
                  tunnel: w437 -> [_ w443]
                  tunnel: w436 -> [_ w442]
                  tunnel: w435 -> [_ w440]
                  tunnel: w434 -> [_ w439]
                  tunnel: w432 -> [_ w438]
                  frame False {
                  }
                  frame True {
                    n267 = local read "STIMULUSINFO \nOFF Count"() -> (w446:u32)
                    n268 = Less?(x=w446, y=w440) -> (x < y?=w444:bool)
                    n269 = Equal?(x=w446, y=0.0) -> (x = y?=w447:bool)
                    n270 = Not(x=w447) -> (.not. x?=w448:bool)
                    n271 = case shown="True" w447 {
                      tunnel: w443 -> [_ w472]
                      tunnel: w442 -> [_ w471]
                      tunnel: w440 -> [_ w470]
                      tunnel: w439 -> [_ w469]
                      tunnel: w438 -> [_ w452]
                      frame False {
                      }
                      frame True {
                        n272 = local read "STIMULUSINFO \nOFF Count"() -> (w466:u32)
                        n273 = local read "Previous Trial: Correct/Incorrect"() -> (w461:bool)
                        n274 = local read "Reinforcement Signal Duration\nFor Incorrect"() -> (w460:dbl)
                        n275 = local read "Reinforcement Signal Duration\nFor correct"() -> (w459:dbl)
                        n276 = local read "TIME Reinforcement OFF"() -> (w468:timestamp)
                        n277 = Less?(x=w466, y=w470) -> (x < y?=w467:bool)
                        n278 = Select(t=w472, s=w461, f=w471) -> (s? t:f=w465:dbl)
                        n279 = local read "ITI"() -> (w464:dbl)
                        n280 = Get Date/Time In Seconds() -> (seconds since 1Jan1904=w463:timestamp)
                        n281 = Add(x=w465, y=w464) -> (x+y=w453:dbl)
                        n282 = Subtract(x=w463, y=w468) -> (x-y=w458:dbl)
                        n283 = Select(t=w459, s=w461, f=w460) -> (s? t:f=w457:dbl)
                        n284 = Add(x=w458, y=w457) -> (x+y=w455:dbl)
                        n285 = Subtract(x=w453, y=w469) -> (x-y=w456:dbl)
                        n286 = Subtract(x=w453, y=w452) -> (x-y=w454:dbl)
                        n287 = In Range and Coerce(upper limit=w453, x=w455, lower limit=w456) -> (In Range?=w462:bool)  [unwired: 1 out]
                        n288 = Less?(x=w455, y=w454) -> (x < y?=w450:bool)
                        n289 = And(x=w462, y=w467) -> (x .and. y?=w451:bool)
                        n290 = And(x=w451, y=w450) -> (x .and. y?=w449:bool)
                        n291 = case shown="True" w449 {
                          frame False {
                            n292 = local write "Stimulation ON?"(FALSE ("Stimulation ON?")) -> ()
                          }
                          frame True {
                            n293 = local write "Stimulation ON?"(TRUE ("Stimulation ON?")) -> ()
                          }
                        }
                      }
                    }
                    n294 = And(x=w448, y=w444) -> (x .and. y?=w445:bool)
                    n295 = case shown="True" w445 {
                      tunnel: w439 -> [_ w483]
                      tunnel: w438 -> [_ w481]
                      frame False {
                      }
                      frame True {
                        n296 = local read "Last STIMULUSINFO OFF"() -> (w485:timestamp)
                        n297 = local read "ISI"() -> (w480:dbl)
                        n298 = Get Date/Time In Seconds() -> (seconds since 1Jan1904=w484:timestamp)
                        n299 = Subtract(x=w484, y=w485) -> (x-y=w478:dbl)
                        n300 = Subtract(x=w480, y=w483) -> (x-y=w482:dbl)
                        n301 = In Range and Coerce(upper limit=w480, x=w478, lower limit=w482) -> (In Range?=w476:bool)  [unwired: 1 out]
                        n302 = Subtract(x=w480, y=w481) -> (x-y=w479:dbl)
                        n303 = Less?(x=w478, y=w479) -> (x < y?=w477:bool)
                        n304 = And(x=w476, y=w477) -> (x .and. y?=w475:bool)
                        n305 = case shown="True" w475 {
                          frame False {
                            n306 = local write "Stimulation ON?"(FALSE ("Stimulation ON?")) -> ()
                          }
                          frame True {
                            n307 = local write "Stimulation ON?"(TRUE ("Stimulation ON?")) -> ()
                          }
                        }
                      }
                    }
                  }
                }
              }
            }
          }
        }
        n308 = Subtract(x=w155, y=w156) -> (x-y=w147:dbl)
        n309 = Less?(x=w147, y=w131) -> (x < y?=w149:bool)
        n310 = Greater?(x=w147, y=0.0) -> (0:w152:bool)
        n311 = event shown="[0] \"ReinfoDur\": Value Change" {
          selector: _ -> [_ _]
          dyn-events: _ -> [_ _]
          timeout: 0 -> [_ _]
          tunnel: w139 -> [w565 _]
          tunnel: w147 -> [w564 _]
          tunnel: [_ 0] -> w146
          tunnel: w137 -> [w563 _]
          tunnel: w131 -> [w562 _]
          event "ReinfoDur": Value Change {
            n312 = event-data() -> ()  [unwired: 1 in, 6 out]
            n313 = flat-sequence {
              tunnel: w565 -> [w570]
              tunnel: w564 -> [w569]
              tunnel: w563 -> [w567]
              tunnel: w562 -> [w566]
              frame #0 {
                n314 = Greater?(x=w569, y=w566) -> (0:w568:bool)
                n315 = local read "REINFORCEMENTINFO \nOFF Count"() -> (w571:u32)
                n316 = case shown="True" w568 {
                  selector: w568 -> [w573 w577]
                  tunnel: w570 -> [_ _]
                  tunnel: [w573 w577] -> _
                  tunnel: w567 -> [_ w575]
                  frame False {
                  }
                  frame True {
                    # "UnSuccessful Trial"
                    n317 = flat-sequence {
                      tunnel: [w595] -> w576
                      tunnel: w576 -> [w598]
                      tunnel: [w604] -> w574
                      frame #0 {
                        n318 = local write "Previous Trial: Correct/Incorrect"(FALSE) -> ()
                      }
                      frame #1 {
                        n319 = local read "# Trials"() -> (w583:u32)
                        n320 = local read "Stimulation Trial"() -> (w582:bool)
                        n321 = local read "# Success"() -> (w585:u32)
                        n322 = Increment(x=w583) -> (x+1=w586:u32)
                        n323 = case shown="True" w582 {
                          frame False {
                            n324 = local read "# Trials: NoSTIM"() -> (w590:u32)
                            n325 = local read "#Success: NoSTIM"() -> (w589:u32)
                            n326 = Increment(x=w590) -> (x+1=w587:u32)
                            n327 = Divide(x=w589, y=w587) -> (x/y=w588:dbl)
                            n328 = local write "# Trials: NoSTIM"(w587) -> ()
                            n329 = local write "% NoSTIM Success"(w588) -> ()
                          }
                          frame True {
                            n330 = local read "# Trials: STIM"() -> (w594:u32)
                            n331 = local read "# Success: STIM"() -> (w591:u32)
                            n332 = Increment(x=w594) -> (x+1=w592:u32)
                            n333 = Divide(x=w591, y=w592) -> (x/y=w593:dbl)
                            n334 = local write "# Trials: STIM"(w592) -> ()
                            n335 = local write "% STIM Success"(w593) -> ()
                          }
                        }
                        n336 = local write "# Trials"(w586) -> ()
                        n337 = Divide(x=w585, y=w586) -> (x/y=w584:dbl)
                        n338 = local write "% Success"(w584) -> ()
                      }
                      frame #2 {
                        n339 = local read "Last Trial End"() -> (w596:timestamp)
                        n340 = Get Date/Time In Seconds() -> (seconds since 1Jan1904=w595:timestamp)
                        n341 = Subtract(x=w595, y=w596) -> (x-y=w597:dbl)
                        n342 = local write "Time Elapsed Since last trial"(w597) -> ()
                      }
                      frame #3 {
                        n343 = local write "Last Trial End"(w598) -> ()
                      }
                      frame #4 {
                        w599 = 0
                        n344 = local write "REINFORCEMENTINFO \nOFF Count"(w599) -> ()
                        n345 = local write "STIMULUSINFO \nON Count"(w599) -> ()
                        n346 = local write "STIMULUSINFO \nOFF Count"(w599) -> ()
                        n347 = local write "REINFORCEMENTINFO \nON Count"(w599) -> ()
                      }
                      frame #5 {
                        n348 = local read "Stimulation Probability"() -> (w607:dbl)
                        n349 = local read "Manually Control Stimulation"() -> (w603:bool)
                        n350 = Subtract(x=1.0, y=w607) -> (x-y=w608:dbl)
                        n351 = Random Number (0-1)() -> (number: 0 to 1=w606:dbl)
                        n352 = Greater Or Equal?(x=w606, y=w608) -> (x >= y?=w604:bool)
                        n353 = case shown="True" w603 {
                          tunnel: [w612 w613] -> w600
                          tunnel: w604 -> [w612 _]
                          frame False {
                          }
                          frame True {
                            n354 = local read "Set StimulationManually, ALWAYS:"() -> (w613:bool)
                          }
                        }
                        n355 = local read "STIM 1 On 1 OFF"() -> (w601:bool)
                        n356 = case shown="True" w601 {
                          tunnel: [w609 w610] -> w602
                          tunnel: w600 -> [w609 _]
                          frame False {
                          }
                          frame True {
                            n357 = local read "Stimulation Trial"() -> (w611:bool)
                            n358 = Not(x=w611) -> (.not. x?=w610:bool)
                          }
                        }
                        n359 = local write "Stimulation Trial"(w602) -> ()
                      }
                    }
                    n360 = case shown="1..6, 8" w575 {
                      tunnel: w574 -> [_ _ w579]
                      frame 0, Default {
                      }
                      frame 1..6, 8 {
                        n361 = local write "Stimulation ON?"(FALSE ("Stimulation ON?")) -> ()
                      }
                      frame 7 {
                        n362 = case shown="True" w579 {
                          frame False {
                          }
                          frame True {
                            n363 = local write "Stimulation ON?"(TRUE ("Stimulation ON?")) -> ()
                          }
                        }
                      }
                    }
                  }
                }
                n364 = Equal?(x=w570, y=w571) -> (x = y?=w572:bool)
                n365 = case shown="True" w572 {
                  tunnel: w567 -> [_ w615]
                  frame False {
                  }
                  frame True {
                    # "If all  reinforcement signals correspond to reward"
                    n366 = flat-sequence {
                      tunnel: [w637] -> w616
                      tunnel: w616 -> [w640]
                      tunnel: [w645] -> w614
                      frame #0 {
                        n367 = local write "Previous Trial: Correct/Incorrect"(TRUE) -> ()
                      }
                      frame #1 {
                        n368 = local read "# Success"() -> (w623:u32)
                        n369 = local read "# Trials"() -> (w622:u32)
                        n370 = local read "Stimulation Trial"() -> (w621:bool)
                        n371 = Increment(x=w623) -> (x+1=w625:u32)
                        n372 = Increment(x=w622) -> (x+1=w626:u32)
                        n373 = Divide(x=w625, y=w626) -> (x/y=w624:dbl)
                        n374 = case shown="False" w621 {
                          frame False {
                            n375 = local read "#Success: NoSTIM"() -> (w630:u32)
                            n376 = local read "# Trials: NoSTIM"() -> (w631:u32)
                            n377 = Increment(x=w630) -> (x+1=w628:u32)
                            n378 = Increment(x=w631) -> (x+1=w627:u32)
                            n379 = Divide(x=w628, y=w627) -> (x/y=w629:dbl)
                            n380 = local write "#Success: NoSTIM"(w628) -> ()
                            n381 = local write "# Trials: NoSTIM"(w627) -> ()
                            n382 = local write "% NoSTIM Success"(w629) -> ()
                          }
                          frame True {
                            n383 = local read "# Success: STIM"() -> (w635:u32)
                            n384 = local read "# Trials: STIM"() -> (w636:u32)
                            n385 = Increment(x=w635) -> (x+1=w633:u32)
                            n386 = Increment(x=w636) -> (x+1=w632:u32)
                            n387 = Divide(x=w633, y=w632) -> (x/y=w634:dbl)
                            n388 = local write "# Success: STIM"(w633) -> ()
                            n389 = local write "# Trials: STIM"(w632) -> ()
                            n390 = local write "% STIM Success"(w634) -> ()
                          }
                        }
                        n391 = local write "# Success"(w625) -> ()
                        n392 = local write "# Trials"(w626) -> ()
                        n393 = local write "% Success"(w624) -> ()
                      }
                      frame #2 {
                        n394 = local read "Last Trial End"() -> (w637:timestamp)
                        n395 = Get Date/Time In Seconds() -> (seconds since 1Jan1904=w638:timestamp)
                        n396 = Subtract(x=w638, y=w637) -> (x-y=w639:dbl)
                        n397 = local write "Time Elapsed Since last trial"(w639) -> ()
                      }
                      frame #3 {
                        n398 = local write "Last Trial End"(w640) -> ()
                      }
                      frame #4 {
                        w641 = 0
                        n399 = local write "STIMULUSINFO \nON Count"(w641) -> ()
                        n400 = local write "REINFORCEMENTINFO \nON Count"(w641) -> ()
                        n401 = local write "STIMULUSINFO \nOFF Count"(w641) -> ()
                        n402 = local write "REINFORCEMENTINFO \nOFF Count"(w641) -> ()
                      }
                      frame #5 {
                        n403 = local read "Stimulation Probability"() -> (w648:dbl)
                        n404 = local read "Manually Control Stimulation"() -> (w650:bool)
                        n405 = Subtract(x=1.0, y=w648) -> (x-y=w649:dbl)
                        n406 = Random Number (0-1)() -> (number: 0 to 1=w647:dbl)
                        n407 = Greater Or Equal?(x=w647, y=w649) -> (x >= y?=w645:bool)
                        n408 = case shown="False" w650 {
                          tunnel: [w654 w655] -> w642
                          tunnel: w645 -> [w654 _]
                          frame False {
                          }
                          frame True {
                            n409 = local read "Set StimulationManually, ALWAYS:"() -> (w655:bool)
                          }
                        }
                        n410 = local read "STIM 1 On 1 OFF"() -> (w644:bool)
                        n411 = case shown="False" w644 {
                          tunnel: [w651 w652] -> w643
                          tunnel: w642 -> [w651 _]
                          frame False {
                          }
                          frame True {
                            n412 = local read "Stimulation Trial"() -> (w653:bool)
                            n413 = Not(x=w653) -> (.not. x?=w652:bool)
                          }
                        }
                        n414 = local write "Stimulation Trial"(w643) -> ()
                      }
                    }
                    n415 = case shown="7" w615 {
                      tunnel: w614 -> [_ _ w618]
                      frame 0, Default {
                      }
                      frame 1..6, 8 {
                        n416 = local write "Stimulation ON?"(FALSE ("Stimulation ON?")) -> ()
                      }
                      frame 7 {
                        n417 = case shown="True" w618 {
                          frame False {
                          }
                          frame True {
                            n418 = local write "Stimulation ON?"(TRUE ("Stimulation ON?")) -> ()
                          }
                        }
                      }
                    }
                  }
                }
              }
              frame #1 {
                n419 = local write "ReinfoDur"(0.0 ("ReinfoDur")) -> ()
              }
              frame #2 {
                n420 = local read "TIME Reinforcement OFF"() -> (w657:timestamp)
                n421 = local write "TIME Reinforcement ON"(w657) -> ()
              }
            }
          }
          event Timeout {
            n422 = event-data() -> ()  [unwired: 1 in, 3 out]
          }
        }
        n423 = And(x=w149, y=w152) -> (x .and. y?=w151:bool)
        n424 = Not(x=w149) -> (.not. x?=w148:bool)
        n425 = call-poly <vilib>:"DAQmx Read.vi"("task/channels in"=w158) -> ("task out"=w157:refnum<k21>, "data"=w135:waveform(dbl)[])  [unwired: 12 in, 1 out]
        n426 = in-place {
          in-place-border: w137 -> [w507]
          in-place-border: w139 -> [w506]
          in-place-border: w138 -> [_]
          in-place-border: w135 -> [w505]
          in-place-border: w134 -> [w504]
          in-place-border: w133 -> [w492]
          in-place-border: w132 -> [w491]
          w494 = u16 0 items=["Falling Edge", "Rising Edge"] ("trigger slope")
          w495 = u16 1 items=["Falling Edge", "Rising Edge"] ("trigger slope")
          # "Hysthersis"
          # "Get rising and falling edges and update the count  STIMINFO and REINFORCEMENTINFO"
          n427 = Equal?(x=w507, y=u16 9) -> (x = y?=w489:bool)
          n428 = Index Array(array=w505, index #1=0 ("index"), index #2=1 ("index")) -> (element #1=w498:waveform(dbl), element #2=w496:waveform(dbl))
          n429 = case shown="True" w489 {
            frame False {
            }
            frame True {
              n430 = local read "Last STIMULATION ON Time"() -> (w511:timestamp)
              n431 = local read "Stimulation Onset time (Before each event )"() -> (w509:dbl)
              n432 = Get Date/Time In Seconds() -> (seconds since 1Jan1904=w512:timestamp)
              n433 = Subtract(x=w512, y=w511) -> (x-y=w510:dbl)
              n434 = Equal?(x=w510, y=w509) -> (x = y?=w508:bool)
              n435 = case shown="True" w508 {
                frame False {
                }
                frame True {
                  n436 = local write "Stimulation ON?"(FALSE ("Stimulation ON?")) -> ()
                }
              }
            }
          }
          n437 = Reciprocal(x=w504) -> (1/x=w493:dbl)
          n438 = in-place {
            in-place-border: [w531] -> w502
            in-place-border: w498 -> [w530]
            in-place-border: w493 -> [w529]
            in-place-border: w495 -> [w527]
            in-place-border: w492 -> [w526]
            in-place-border: w491 -> [w525]
            in-place-border: [w524] -> w503
            in-place-border: w494 -> [w523]
            # "STIMULUSINFO THRESHOLD"
            n439 = Bundle By Name(cluster=w530, "dt"=w529) -> (w528:waveform(dbl))
            n440 = call-poly <vilib>:"Basic Level Trigger Detection.vi"("signal in"=w528, "level"=w526, "hysteresis"=w525, "trigger slope"=w527) -> ("trigger detected?"=w524:bool)  [unwired: 9 in, 2 out]
            n441 = call-poly <vilib>:"Basic Level Trigger Detection.vi"("signal in"=w528, "level"=w526, "hysteresis"=w525, "trigger slope"=w523) -> ("trigger detected?"=w531:bool)  [unwired: 9 in, 2 out]
          }
          n442 = in-place {
            in-place-border: [w522] -> w500
            in-place-border: w493 -> [w521]
            in-place-border: w496 -> [w520]
            in-place-border: w495 -> [w519]
            in-place-border: w492 -> [w517]
            in-place-border: w491 -> [w516]
            in-place-border: w494 -> [w515]
            in-place-border: [w514] -> w501
            # "REINFORCEMENTINFO THRESHOLD"
            n443 = Bundle By Name(cluster=w520, "dt"=w521) -> (w518:waveform(dbl))
            n444 = call-poly <vilib>:"Basic Level Trigger Detection.vi"("signal in"=w518, "level"=w517, "hysteresis"=w516, "trigger slope"=w519) -> ("trigger detected?"=w522:bool)  [unwired: 9 in, 2 out]
            n445 = call-poly <vilib>:"Basic Level Trigger Detection.vi"("signal in"=w518, "level"=w517, "hysteresis"=w516, "trigger slope"=w515) -> ("trigger detected?"=w514:bool)  [unwired: 9 in, 2 out]
          }
          n446 = case shown="True" w503 {
            frame False {
            }
            frame True {
              # "StimInfo rising edge trigger"
              n447 = local read "STIMULUSINFO \nON Count"() -> (w559:u32)
              n448 = Increment(x=w559) -> (x+1=w560:u32)
              n449 = local write "STIMULUSINFO \nON Count"(w560) -> ()
            }
          }
          n450 = case shown="True" w502 {
            tunnel: w507 -> [_ w540]
            tunnel: w506 -> [_ w539]
            frame False {
            }
            frame True {
              # "StimInfo Falling edge trigger"
              n451 = flat-sequence {
                tunnel: [w553] -> w538
                tunnel: [w555] -> w541
                tunnel: w541 -> [w558]
                frame #0 {
                  # "Update Stimulus OFF Count"
                  n452 = local read "STIMULUSINFO \nOFF Count"() -> (w554:u32)
                  n453 = Increment(x=w554) -> (x+1=w553:u32)
                  n454 = local write "STIMULUSINFO \nOFF Count"(w553) -> ()
                }
                frame #1 {
                  # "Get StimulusOff time"
                  n455 = local read "Last STIMULUSINFO OFF"() -> (w557:timestamp)
                  n456 = Get Date/Time In Seconds() -> (seconds since 1Jan1904=w555:timestamp)
                  n457 = Subtract(x=w555, y=w557) -> (x-y=w556:dbl)
                  n458 = local write "Time Elapsed since last event Offset"(w556) -> ()
                }
                frame #2 {
                  # "Update Value"
                  n459 = local write "Last STIMULUSINFO OFF"(w558) -> ()
                }
              }
              n460 = case shown="1..3" w540 {
                tunnel: w539 -> [_ _ w545 w550]
                tunnel: w538 -> [_ _ w543 w551]
                frame 0, Default {
                }
                frame 1..3 {
                  n461 = local write "Stimulation ON?"(FALSE ("Stimulation ON?")) -> ()
                }
                frame 4 {
                  n462 = Equal?(x=w543, y=w545) -> (x = y?=w544:bool)
                  n463 = case shown="True" w544 {
                    frame False {
                    }
                    frame True {
                      n464 = local write "Stimulation ON?"(FALSE ("Stimulation ON?")) -> ()
                    }
                  }
                }
                frame 5 {
                  n465 = Multiply(x=w550, y=u16 2) -> (x*y=w548:u16)
                  n466 = Equal?(x=w551, y=w548) -> (x = y?=w547:bool)
                  n467 = case shown="True" w547 {
                    frame False {
                    }
                    frame True {
                      n468 = local write "Stimulation ON?"(FALSE ("Stimulation ON?")) -> ()
                    }
                  }
                }
              }
            }
          }
          n469 = case shown="True" w500 {
            frame False {
            }
            frame True {
              # "ReinforcementInfo rising edge trigger"
              n470 = Get Date/Time In Seconds() -> (seconds since 1Jan1904=w535:timestamp)
              n471 = local read "REINFORCEMENTINFO \nON Count"() -> (w536:u32)
              n472 = local write "TIME Reinforcement ON"(w535) -> ()
              n473 = Increment(x=w536) -> (x+1=w537:u32)
              n474 = local write "REINFORCEMENTINFO \nON Count"(w537) -> ()
            }
          }
          n475 = case shown="True" w501 {
            frame False {
            }
            frame True {
              # "ReinforcementInfo Falling edge trigger"
              n476 = Get Date/Time In Seconds() -> (seconds since 1Jan1904=w532:timestamp)
              n477 = local read "REINFORCEMENTINFO \nOFF Count"() -> (w533:u32)
              n478 = local write "TIME Reinforcement OFF"(w532) -> ()
              n479 = Increment(x=w533) -> (x+1=w534:u32)
              n480 = local write "REINFORCEMENTINFO \nOFF Count"(w534) -> ()
            }
          }
        }
        n481 = case shown="True" w148 {
          tunnel: w147 -> [_ w488]
          tunnel: w146 -> [_ _]
          frame False {
          }
          frame True {
            # "Unsuccessful Trial"
            n482 = property on="ReinfoDur" class="DigNum (strict)"("Val(Sgnl)"=w488) -> ()  [unwired: 2 in, 2 out]
          }
        }
        n483 = case shown="True" w151 {
          tunnel: w147 -> [_ w561]
          tunnel: w146 -> [_ _]
          frame False {
          }
          frame True {
            # "Successful trial"
            n484 = property on="ReinfoDur" class="DigNum (strict)"("Val(Sgnl)"=w561) -> ()  [unwired: 2 in, 2 out]
          }
        }
      }
      n485 = call "Convert from Dynamic Data"("Dynamic Data Type"=w81) -> ("Array"=w80:bool[])  [unwired: 3 in]
      n486 = while {
        tunnel: w80 -> [w104]
        tunnel: w79 -> [w103]
        tunnel: [w101] -> w76
        tunnel: w73 -> [w99]
        stop <- w102 stop-if-true
        # "Generate TTL Pulse if Stimulation ON? is true"
        n487 = call <vilib>:"High Resolution Polling Wait.vi"("seconds to wait"=w99) -> ()  [unwired: 10 in, 1 out]
        n488 = local read "Stimulation ON?"() -> (w105:bool)
        n489 = case shown="False" w105 {
          tunnel: w104 -> [_ w110]
          tunnel: [0.0 ("f") w108] -> w100
          frame False {
            (unwired) FALSE
            # "Reset the stimulation pulse counter"
            n490 = local write "Stimulation Pulse Counter"(u64 0 ("Stimulation Pulse Counter")) -> ()
          }
          frame True {
            # "Get the TTL index it and write to Digital out channel"
            n491 = flat-sequence {
              tunnel: w110 -> [w115]
              tunnel: [w114] -> w109
              tunnel: [w111] -> w108
              tunnel: [w119] -> _
              tunnel: w109 -> [w119]
              frame #0 {
                n492 = local read "Stimulation Pulse Counter"() -> (w116:u64)
                n493 = Index Array(array=w115, index=w116) -> (element=w114:bool)
                n494 = Select(t=5.0, s=w114, f=0.0) -> (s? t:f=w111:dbl)
              }
              frame #1 {
                n495 = local read "Stimulation Pulse Counter"() -> (w118:u64)
                n496 = Increment(x=w118) -> (x+1=w117:u64)
                n497 = local write "Stimulation Pulse Counter"(w117) -> ()
              }
            }
          }
        }
        n498 = call-poly <vilib>:"DAQmx Write.vi"("task/channels in"=w103, "data"=w100) -> ("task out"=w101:refnum<k21>)  [unwired: 11 in, 2 out]
        n499 = local read "stop"() -> (w102:bool)
      }
      n500 = call <vilib>:"DAQmx Stop Task.vi"("task/channels in"=w76) -> ("task out"=w78:refnum<k21>, "error out"=w77:errorcluster)  [unwired: 13 in]
      n501 = call <vilib>:"DAQmx Clear Task.vi"("task in"=w78, "error in"=w77) -> ()  [unwired: 13 in, 1 out]
      n502 = Stop(stop? (T)=w94) -> ()
      n503 = call <vilib>:"DAQmx Stop Task.vi"("task/channels in"=w97) -> ("task out"=w98:refnum<k21>, "error out"=w95:errorcluster)  [unwired: 13 in]
      n504 = call <vilib>:"DAQmx Clear Task.vi"("task in"=w98, "error in"=w95) -> ()  [unwired: 13 in, 1 out]
    }
  }
